vi "Configure Digital Pattern Address.vi"(4 "Custom Stop Address (2)":i32=2 min=1 max=262144, 5 "Custom Start Address (1)":i32=1 min=1 max=262144, 6 "Stop Adrress (Maximum)":enum16{"Minimum", "Maximum", "Custom"}(ring)=enum."Maximum", 7 "Start Adrress (Minimum)":enum16{"Minimum", "Maximum", "Custom"}(ring), 8 "error in (no error)":errorcluster, 11 "VISA resource name":refnum<visa-resource-name>) -> (0 "error out":errorcluster, 3 "VISA resource name out":refnum<visa-resource-name>)   [LabVIEW 2017, in "Keithley 3390.lvlib"]
doc: "Configures the Start and Stop Address of the digital pattern."
uses:
  Keithley 3390.lvlib
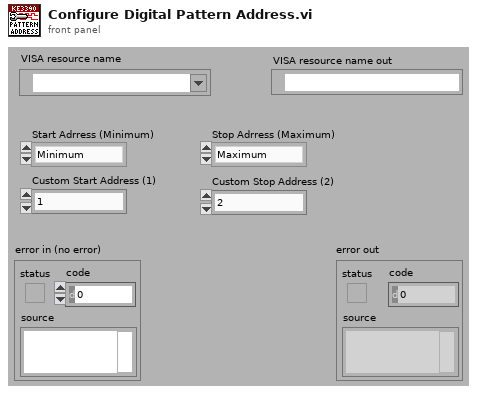
[diagram p1: front panel]
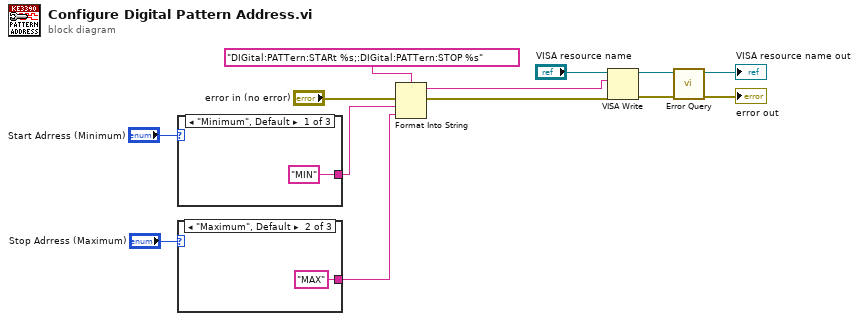
[diagram p0: block diagram]
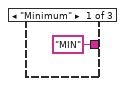
[diagram p2: hidden frame]
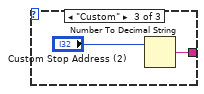
[diagram p3: hidden frame]
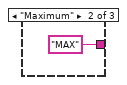
[diagram p4: hidden frame]
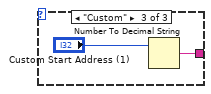
[diagram p5: hidden frame]
diagram:
  n1 = case shown="\"Minimum\", Default" "Start Adrress (Minimum)" {
    tunnel: ["MIN" "MAX" w16] -> w8
    frame "Minimum", Default {
    }
    frame "Maximum" {
    }
    frame "Custom" {
      n2 = Number To Decimal String(number="Custom Start Address (1)") -> (decimal integer string=w16:string)  [unwired: 1 in]
    }
  }
  n3 = case shown="\"Maximum\", Default" "Stop Adrress (Maximum)" {
    tunnel: ["MIN" "MAX" w20] -> w7
    frame "Minimum" {
    }
    frame "Maximum", Default {
    }
    frame "Custom" {
      n4 = Number To Decimal String(number="Custom Stop Address (2)") -> (decimal integer string=w20:string)  [unwired: 1 in]
    }
  }
  n5 = Format Into String(format string="DIGital:PATTern:STARt %s;:DIGital:PATTern:STOP %s", error in="error in (no error)", w8, w7) -> (resulting string=w5:string, error out=w6:errorcluster)  [unwired: 1 in]
  n6 = VISA Write(VISA resource name="VISA resource name", write buffer=w5, error in (no error)=w6) -> (VISA resource name out=w3:refnum<visa-resource-name>, error out=w4:errorcluster)  [unwired: 1 out]
  n7 = call "Error Query.vi"("error in (no error)"=w4, "VISA resource name"=w3) -> ("error out"=→"error out":errorcluster, "VISA resource name out"=→"VISA resource name out":refnum<visa-resource-name>)  [unwired: 6 in, 2 out]
